vi "Test#CMDExecute.vi"(3 "ProgramRef":refnum<vi>, 4 "Command":string[](array[string]), 5 "ThreadsQueue":refnum<queue>[](array[refnum]), 6 "ThreadNo.":u32, 7 "ThreadModReceive":refnum<queue>[](array[refnum]), 8 "StackIn":cluster{"Program":i32, "Prog Index":i32}[](array[cluster]), 9 "ThreadInfoIn":T1) -> (0 "StackOut":cluster{"Program":i32, "Prog Index":i32}[](array[cluster]), 1 "ThreadInfoOut":T1, 2 "ErrorCode":string)   [LabVIEW 2019]
uses:
  MainFrame/Global.vi
panel:
  out "KeyFind?":bool[](array[boolean])
  out "KeyValues":string[](array[string])
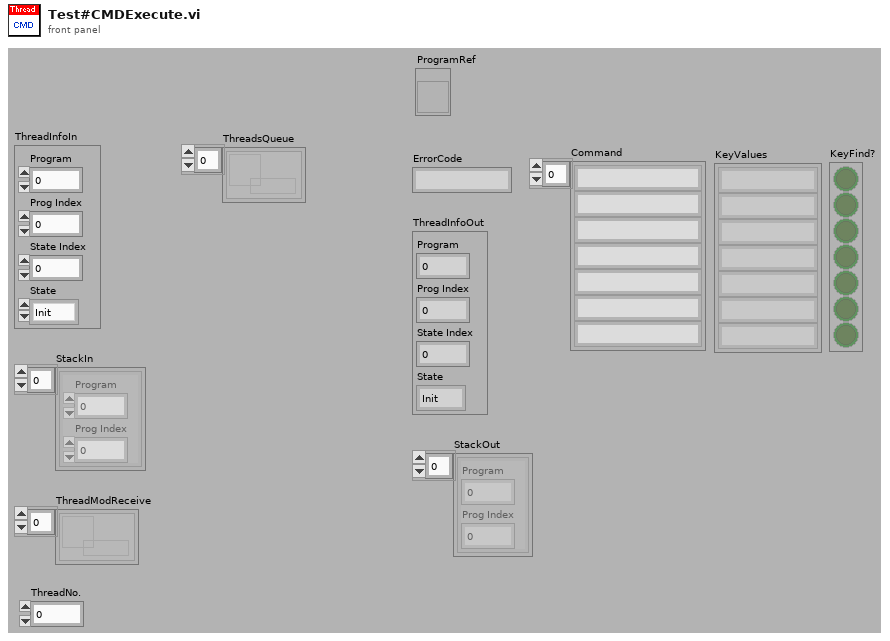
[diagram p1: front panel]
types:
  T1 = cluster{"Program":i32, "Prog Index":i32, "State Index":i32, "State":enum16{"Init", "Idle", "Auto Start", "Auto Running", "Step Start", "Step Running", "Suspend", "Restart", "Stop", "Reset"}}
  T2 = cluster{"指令":string, "代碼":string, "參數長度":i32, "乘數":dbl, "加數":dbl}[]
  T3 = cluster{"Command":string, "Parameter":string, "queue out":refnum<queue>}
  T4 = cluster{"指令":string, "代碼":string, "參數長度":i32, "乘數":dbl, "加數":dbl}[][]
  T5 = cluster{"指令":string, "代碼":string, "參數長度":i32, "乘數":dbl, "加數":dbl}
  T6 = enum16{"Init", "Idle", "Auto Start", "Auto Running", "Step Start", "Step Running", "Suspend", "Restart", "Stop", "Reset"}
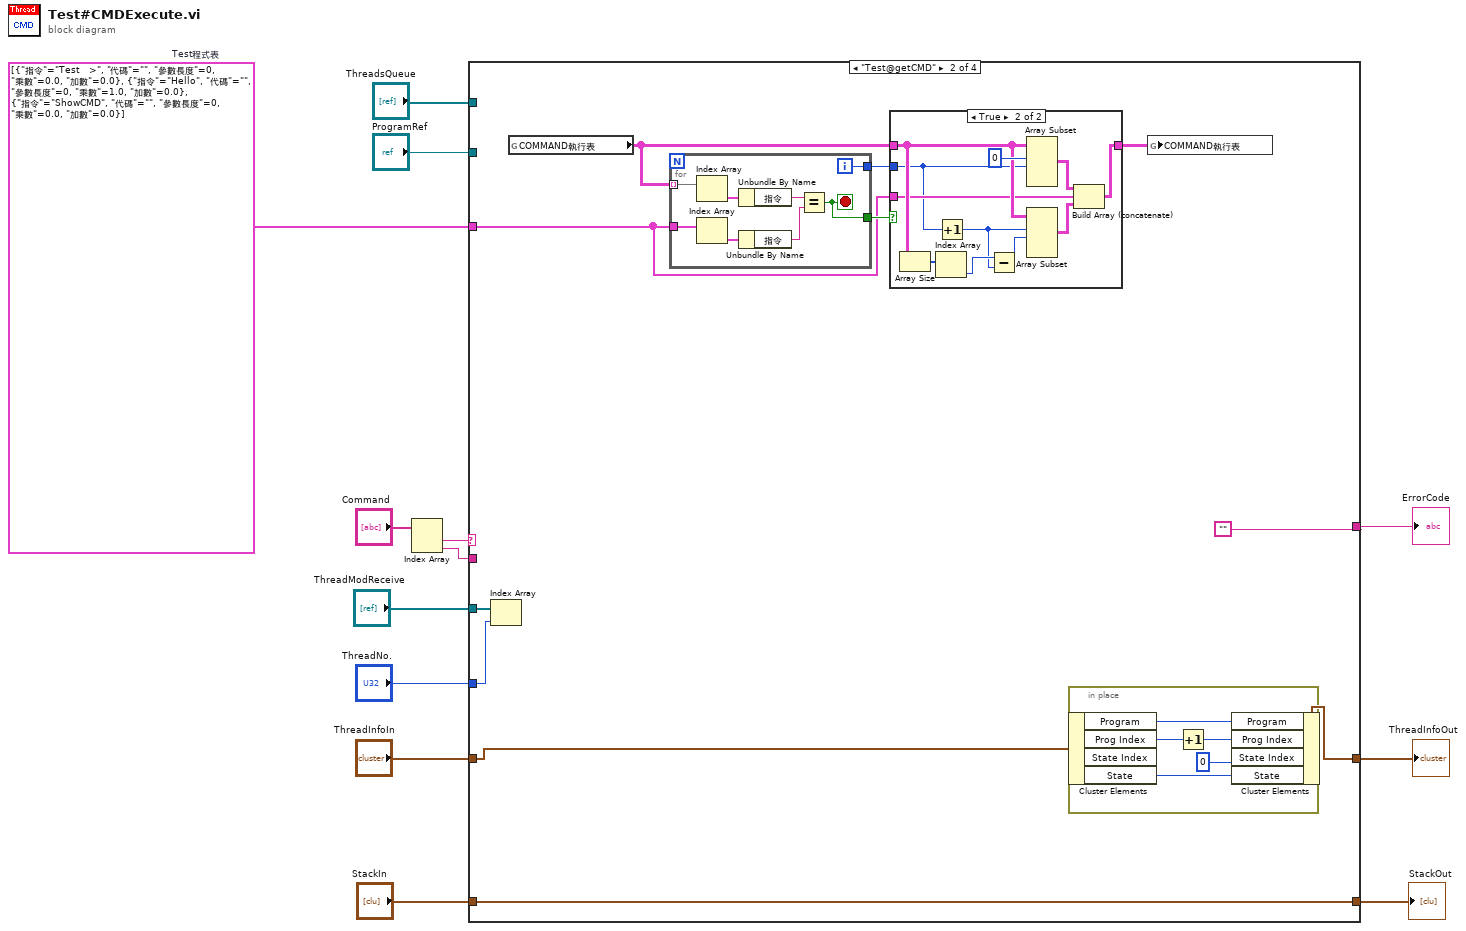
[diagram p0: block diagram]
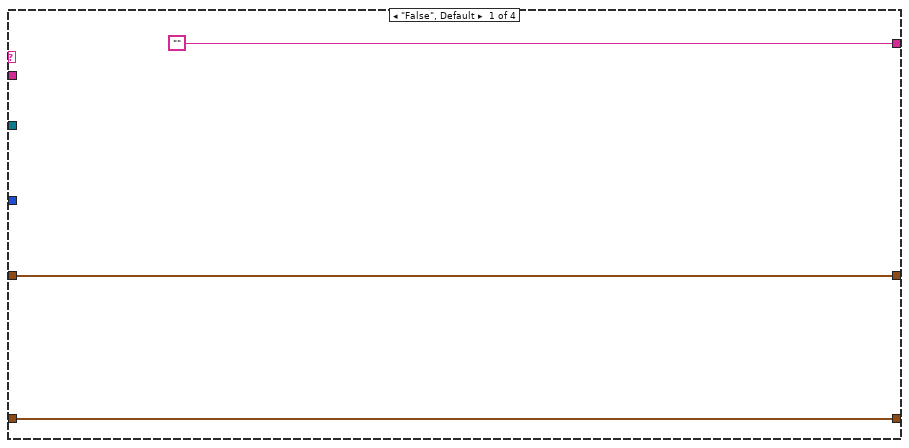
[diagram p2: hidden frame]
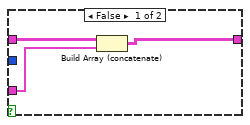
[diagram p3: hidden frame]
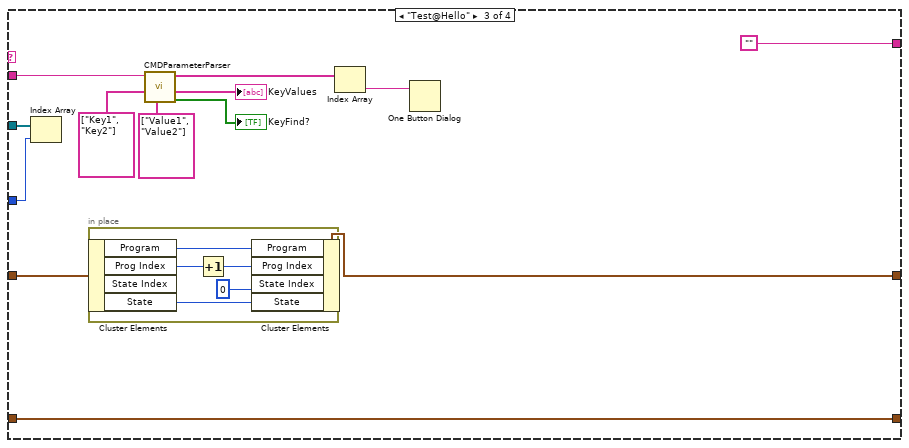
[diagram p4: hidden frame]
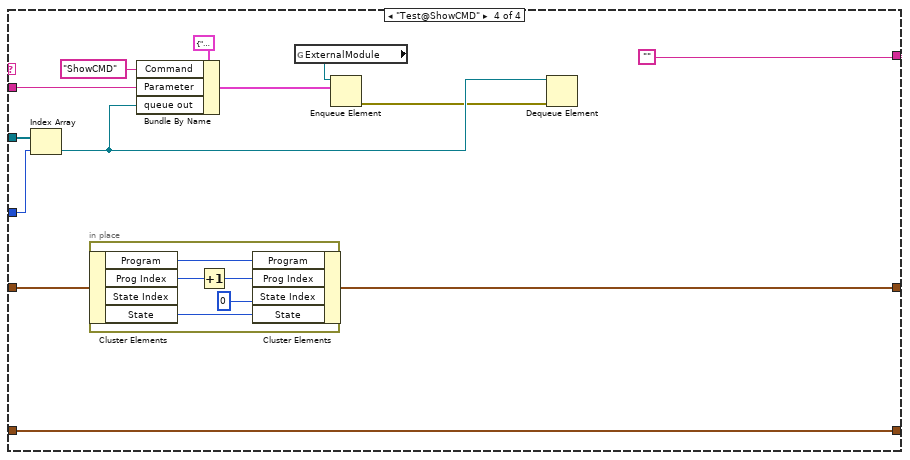
[diagram p5: hidden frame]
diagram:
  w2 = T2 [{"指令"="Test   >", "代碼"="", "參數長度"=0, "乘數"=0.0, "加數"=0.0}, {"指令"="Hello", "代碼"="", "參數長度"=0, "乘數"=1.0, "加數"=0.0}, {"指令"="ShowCMD", "代碼"="", "參數長度"=0, "乘數"=0.0, "加數"=0.0}]  # Test程式表
  n1 = Index Array(array="Command") -> (element #1=w10:string, element #2=w8:string)  [unwired: 2 in]
  n2 = case shown="\"Test@getCMD\"" w10 {
    tunnel: "ThreadModReceive" -> [_ w27 w67 w85]
    tunnel: [w16 w25 w65 w83] -> w5
    tunnel: "ThreadInfoIn" -> [w16 w24 w64 w82]
    tunnel: "ThreadNo." -> [_ w26 w66 w84]
    tunnel: w8 -> [_ _ w61 w79]
    tunnel: "ThreadsQueue" -> [_ _ _ _]
    tunnel: ["" "" "" ""] -> w11
    tunnel: [w14 w23 w63 w81] -> w12
    tunnel: "StackIn" -> [w14 w23 w63 w81]
    tunnel: w2 -> [_ w19 _ _]
    tunnel: "ProgramRef" -> [_ _ _ _]
    frame "False", Default {
    }
    frame "Test@getCMD" {
      n3 = Index Array(array=w27, index=w26) -> ()  [unwired: 1 out]
      n4 = global read "Global.vi" "COMMAND執行表"() -> (w18:T4)
      n5 = for {
        tunnel: w18 -> [w47] mode=indexing
        tunnel: w19 -> [w48]
        tunnel: [w43] -> w20
        tunnel: [w42] -> w21
        i -> [w43]
        stop <- w42 stop-if-true
        n6 = Index Array(array=w47) -> (element=w49:T5)  [unwired: 1 in]
        n7 = Index Array(array=w48) -> (element=w46:T5)  [unwired: 1 in]
        n8 = Unbundle By Name(w49) -> ("指令"=w45:string)
        n9 = Unbundle By Name(w46) -> ("指令"=w44:string)
        n10 = Equal?(x=w45, y=w44) -> (x = y?=w42:bool)
      }
      n11 = case shown="True" w21 {
        tunnel: w20 -> [_ w32]
        tunnel: w19 -> [w29 w35]
        tunnel: w18 -> [w30 w40]
        tunnel: [w28 w33] -> w17
        frame False {
          n12 = Build Array (concatenate)(w30, w29) -> (w28:T4)
        }
        frame True {
          n13 = Array Size(array=w40) -> (size(s)=w39:i32[])
          n14 = Index Array(array=w39) -> (element=w38:i32)  [unwired: 1 in]
          n15 = Increment(x=w32) -> (x+1=w31:i32)
          n16 = Subtract(x=w38, y=w31) -> (x-y=w37:i32)
          n17 = Array Subset(array=w40, index (row)=0 ("index"), length (row)=w32) -> (w36:T4)  [unwired: 2 in]
          n18 = Array Subset(array=w40, index (row)=w31, length (row)=w37) -> (w34:T4)  [unwired: 2 in]
          n19 = Build Array (concatenate)(w36, w35, w34) -> (w33:T4)
        }
      }
      n20 = in-place {
        n21 = in-place-cluster #1(w24) -> ("Program"=w54:i32, "Prog Index"=w52:i32, "State"=w50:T6)  [unwired: 1 out]
        n22 = Increment(x=w52) -> (x+1=w53:i32)
        n23 = in-place-cluster #1("Program"=w54, "Prog Index"=w53, "State Index"=0, "State"=w50) -> (w25:T1)
      }
      n24 = global write "Global.vi" "COMMAND執行表"(w17) -> ()
    }
    frame "Test@Hello" {
      n25 = Index Array(array=w67, index=w66) -> ()  [unwired: 1 out]
      n26 = in-place {
        n27 = in-place-cluster #2(w64) -> ("Program"=w72:i32, "Prog Index"=w70:i32, "State"=w68:T6)  [unwired: 1 out]
        n28 = Increment(x=w70) -> (x+1=w71:i32)
        n29 = in-place-cluster #2("Program"=w72, "Prog Index"=w71, "State Index"=0, "State"=w68) -> (w65:T1)
      }
      n30 = call "CMDParameterParser.vi"("DeafultValues"=string[] ["Value1", "Value2"] ("RequiredKeys"), "RequiredKeys"=string[] ["Key1", "Key2"], "CMDParameter"=w61) -> ("KeyFind?"=→"KeyFind?":bool[], "KeyValues"=→"KeyValues":string[], "Input"=w60:string[])  [unwired: 6 in]
      n31 = Index Array(array=w60) -> (element=w55:string)  [unwired: 1 in]
      n32 = One Button Dialog(message=w55) -> ()  [unwired: 1 in, 1 out]
    }
    frame "Test@ShowCMD" {
      n33 = Index Array(array=w85, index=w84) -> (element=w78:refnum<queue>)
      n34 = in-place {
        n35 = in-place-cluster #3(w82) -> ("Program"=w90:i32, "Prog Index"=w88:i32, "State"=w86:T6)  [unwired: 1 out]
        n36 = Increment(x=w88) -> (x+1=w89:i32)
        n37 = in-place-cluster #3("Program"=w90, "Prog Index"=w89, "State Index"=0, "State"=w86) -> (w83:T1)
      }
      n38 = Bundle By Name(cluster=T3 {"Command"="", "Parameter"="", "queue out"=refnum} ("CMD"), "Command"="ShowCMD", "Parameter"=w79, "queue out"=w78) -> (w75:T3)
      n39 = global read "Global.vi" "ExternalModule"() -> (w77:refnum<queue>)
      n40 = Enqueue Element(queue=w77, element=w75) -> (error out=w73:errorcluster)  [unwired: 2 in, 2 out]
      n41 = Dequeue Element(queue=w78, error in (no error)=w73) -> ()  [unwired: 1 in, 4 out]
    }
  }
  "StackOut" <- w12
  "ErrorCode" <- w11
  "ThreadInfoOut" <- w5
